vi "check_start_conditions.vi"(4 "FIFO overflow?":bool, 6 "stop at FIFO overflow?":bool, 7 "converter box version":i16=1 min=1 max=2, 9 "already acquiring?":bool, 10 "in triggered mode?":bool, 11 "acquire":bool) -> (2 "acquire?":bool)   [LabVIEW 2010]
uses:
  <vilib>/eio/EIONode/EIONode.xnode
  <vilib>/rvi/eio/nirviEIOImplementation/nirviEIOImplementation.xnode
  <vilib>/rvi/eio/common/nirviEmuClasses.ctl
  <vilib>/rvi/eio/common/nirviEmuTemplateMethod_noerrors.vi
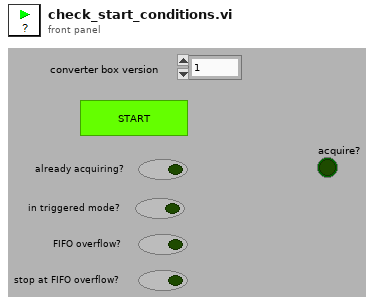
[diagram p1: front panel]
types:
  T1 = typedef "nirviEmuClasses.ctl" = enum16{"IO Read", "IO Write", "Method", "Property Read", "Property Write"}
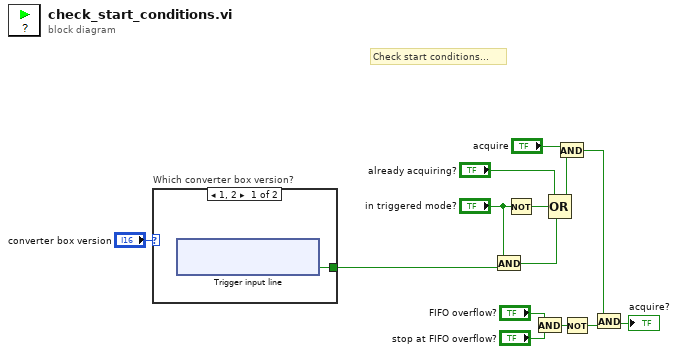
[diagram p0: block diagram]
diagram:
  # "Check start conditions..."
  n1 = case "Which converter box version?" shown="1, 2" "converter box version" {
    tunnel: [w15 _] -> w11
    frame 1, 2 {
      n2 = xnode "Trigger input line"() -> ("Connector0/DIO34"=w15:bool)  [unwired: 1 in, 1 out]
    }
    frame Default {
    }
  }
  n3 = And(x="in triggered mode?", y=w11) -> (x .and. y?=w9:bool)
  n4 = Not(x="in triggered mode?") -> (.not. x?=w12:bool)
  n5 = And(x="FIFO overflow?", y="stop at FIFO overflow?") -> (x .and. y?=w6:bool)
  n6 = Compound Arithmetic op=OR("already acquiring?", w12, w9) -> (w14:bool)
  n7 = And(x="acquire", y=w14) -> (x .and. y?=w4:bool)
  n8 = Not(x=w6) -> (.not. x?=w5:bool)
  n9 = And(x=w4, y=w5) -> (x .and. y?=→"acquire?":bool)
